vi "Menu Selection-to-Listbox Item.vi"(8 "error in (no error)":errorcluster, 10 "String":string, 11 "Menu Refnum":refnum<k9>) -> (0 "error out":errorcluster)   [LabVIEW 2023]
panel:
  out "Numeric":i32
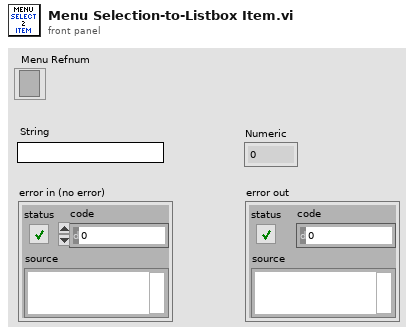
[diagram p1: front panel]
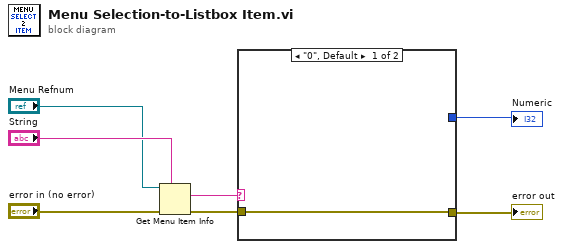
[diagram p0: block diagram]
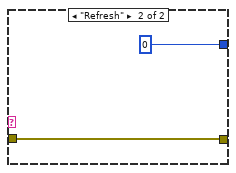
[diagram p2: hidden frame]
diagram:
  n1 = Get Menu Item Info(7:"String", 8:"error in (no error)", 11:"Menu Refnum") -> (0:w1:errorcluster, 2:w5:string)  [unwired: 5 out]
  n2 = case shown="\"0\", Default" w5 {
    tunnel: w1 -> [w8 w10]
    tunnel: [w8 w10] -> w7
    tunnel: [_ 0] -> w3
    frame "0", Default {
    }
    frame "Refresh" {
    }
  }
  "error out" <- w7
  "Numeric" <- w3
